vi "auton_exec.vi"(8 "test (devel auton)":bool, 9 "reinit":bool, 10 "bus_inputs":T1, 11 "bus_state":T2) -> (2 "bus_inputs out":T1, 3 "bus_state out":T2)   [LabVIEW 2013]
uses:
  structures/bus_state.ctl
  structures/bus_state_drivetrain.ctl
  structures/bus_state_collector.ctl
  collector/collector_shot_cal.ctl
  structures/bus_inputs.ctl
  auto_data.vi
  scriptlib/NAV_DRIVE_STOP.vi
  scriptlib/FIRE.vi
  scriptlib/WAIT_FOR_GUN.vi
  scriptlib/WAIT.vi
  scriptlib/NAV_DRIVE_STRAIGHT.vi
  scriptlib/CLOSE.vi
  scriptlib/WAIT_FOR_BALL.vi
  scriptlib/CAL_SET_SHOT_AUTON_1.vi
  scriptlib/SUCK.vi
  scriptlib/NOSUCK.vi
panel:
  out "autontime":u32
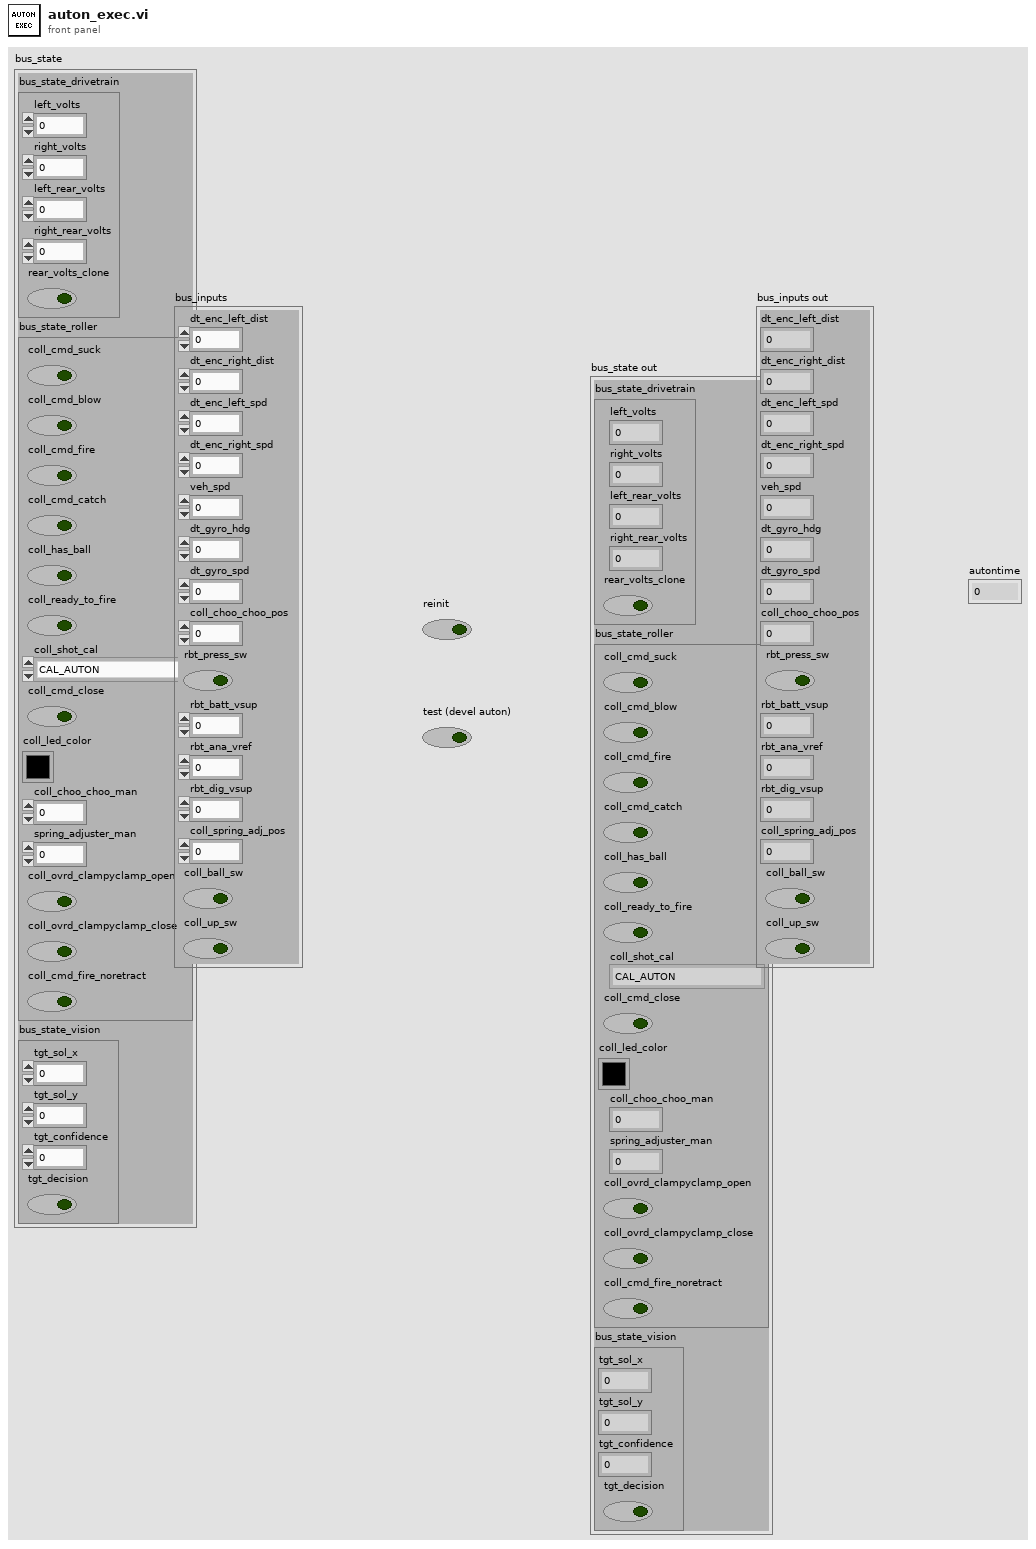
[diagram p1: front panel]
types:
  T1 = typedef "bus_inputs.ctl" = cluster{"dt_enc_left_dist":sgl, "dt_enc_right_dist":sgl, "dt_enc_left_spd":sgl, "dt_enc_right_spd":sgl, "veh_spd":sgl, "dt_gyro_hdg":sgl, "dt_gyro_spd":sgl, "coll_choo_choo_pos":sgl, "rbt_press_sw":bool, "rbt_batt_vsup":sgl, "rbt_ana_vref":dbl, "rbt_dig_vsup":dbl, "coll_spring_adj_pos":sgl, "coll_ball_sw":bool, "coll_up_sw":bool}
  T2 = typedef "bus_state.ctl" = cluster{"bus_state_drivetrain":T3, "bus_state_roller":T4, "bus_state_vision":cluster{"tgt_sol_x":dbl, "tgt_sol_y":dbl, "tgt_confidence":dbl, "tgt_decision":bool}}
  T3 = typedef "bus_state_drivetrain.ctl" = cluster{"left_volts":sgl, "right_volts":sgl, "left_rear_volts":sgl, "right_rear_volts":sgl, "rear_volts_clone":bool}
  T4 = typedef "bus_state_collector.ctl" = cluster{"coll_cmd_suck":bool, "coll_cmd_blow":bool, "coll_cmd_fire":bool, "coll_cmd_catch":bool, "coll_has_ball":bool, "coll_ready_to_fire":bool, "coll_shot_cal":T5, "coll_cmd_close":bool, "coll_led_color":u32, "coll_choo_choo_man":sgl, "spring_adjuster_man":sgl, "coll_ovrd_clampyclamp_open":bool, "coll_ovrd_clampyclamp_close":bool, "coll_cmd_fire_noretract":bool}
  T5 = typedef "collector_shot_cal.ctl" = enum16{"CAL_AUTON", "CAL_CLOSE", "CAL_MID", "CAL_FAR", "NOT_SAFE_TO_ACTUATE"}
  T6 = typedef "vi_execute.ctl" = cluster{"arguments":string[], "command":string, "refnum valid check":bool, "vi_ind":u8}
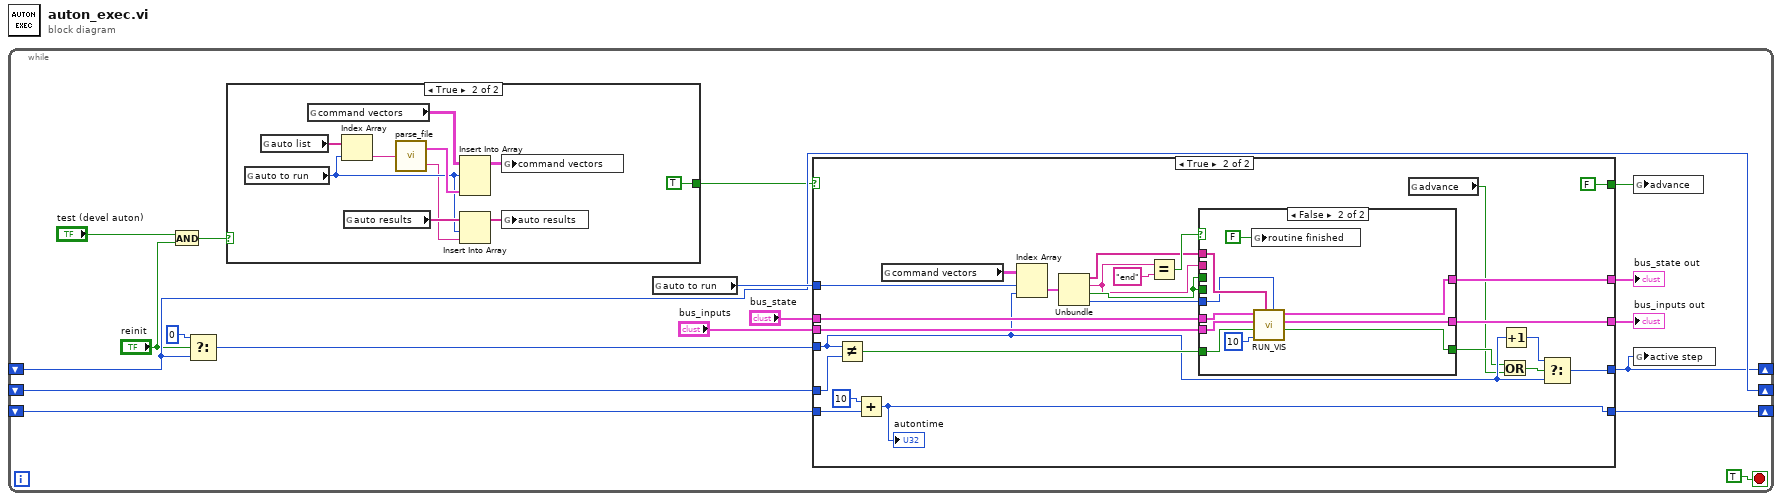
[diagram p0: block diagram]
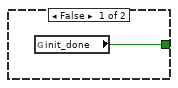
[diagram p2: hidden frame]
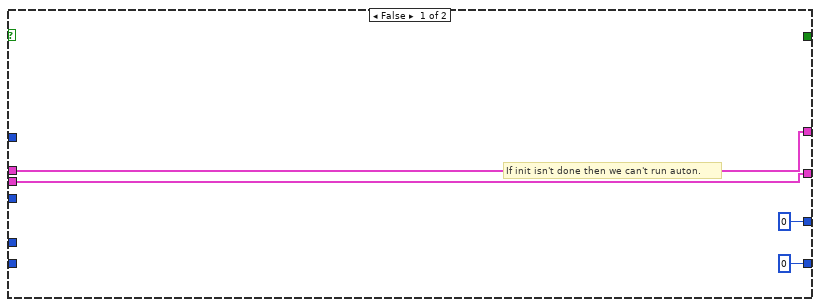
[diagram p3: hidden frame]
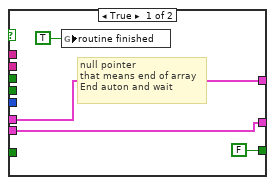
[diagram p4: hidden frame]
diagram:
  n1 = while {
    shift-right: [w2] -> _
    shift-left: _ -> [w11]
    shift-right: [w11] -> _
    shift-left: _ -> [w12]
    shift-right: [w4] -> _
    shift-left: _ -> [w5]
    stop <- TRUE stop-if-true
    n2 = And(x="test (devel auton)", y="reinit") -> (x .and. y?=w6:bool)
    n3 = Select(t=u16 0, s="reinit", f=w11) -> (s? t:f=w10:u16)
    n4 = case shown="True" w6 {
      tunnel: [w19 TRUE ("init_done")] -> w3
      frame False {
        n5 = global read "auto_data.vi" "init_done"() -> (w19:bool)
      }
      frame True {
        n6 = global read "auto_data.vi" "auto to run"() -> (w22:u8)
        n7 = global read "auto_data.vi" "auto list"() -> (w29:string[])
        n8 = global read "auto_data.vi" "command vectors"() -> (w27:T6[][])
        n9 = Index Array(array=w29, index=w22) -> (element=w28:string)
        n10 = global read "auto_data.vi" "auto results"() -> (w24:string[])
        n11 = call "parse_file.vi"("File Name With Extension"=w28) -> ("command vector"=w26:T6[], "file_status"=w21:string)
        n12 = Insert Into Array(array=w27, index (row)=w22, new element=w26) -> (w25:T6[][])  [unwired: 1 in]
        n13 = Insert Into Array(array=w24, index=w22, new element=w21) -> (w23:string[])
        n14 = global write "auto_data.vi" "command vectors"(w25) -> ()
        n15 = global write "auto_data.vi" "auto results"(w23) -> ()
      }
    }
    n16 = global read "auto_data.vi" "auto to run"() -> (w17:u8)
    n17 = case shown="True" w3 {
      tunnel: w17 -> [_ w43]
      tunnel: w10 -> [_ w42]
      tunnel: "bus_state" -> [w33 w54]
      tunnel: [w33 w56] -> w15
      tunnel: [w32 w55] -> w14
      tunnel: "bus_inputs" -> [w32 w53]
      tunnel: [u16 0 w50] -> w2
      tunnel: w12 -> [_ w52]
      tunnel: w5 -> [_ w48]
      tunnel: [u32 0 w47] -> w4
      tunnel: [_ FALSE] -> w1
      frame False {
        # "If init isn't done then we can't run auton."
      }
      frame True {
        n18 = Not Equal?(x=w42, y=w52) -> (x != y?=w51:bool)
        n19 = Add(x=u32 10, y=w48) -> (x+y=w47:u32)
        "autontime" <- w47
        n20 = global read "auto_data.vi" "command vectors"() -> (w58:T6[][])
        n21 = Index Array(array=w58, index (row)=w43, index (col)=w42) -> (element=w57:T6)
        n22 = Unbundle(w57) -> ("arguments"=w44:string[], "command"=w35:string, "refnum valid check"=w37:bool, "vi_ind"=w36:u8)
        n23 = Equal?(x=w35, y="end") -> (x = y?=w45:bool)
        n24 = case shown="False" w45 {
          tunnel: w44 -> [_ w70]
          tunnel: w35 -> [_ _]
          tunnel: [w62 w66] -> w56
          tunnel: [w60 w65] -> w55
          tunnel: w54 -> [w62 w71]
          tunnel: w53 -> [w60 w67]
          tunnel: w51 -> [_ w68]
          tunnel: [FALSE ("Done") w64] -> w40
          tunnel: w37 -> [_ _]
          tunnel: w37 -> [_ _]
          tunnel: w36 -> [_ w63]
          frame True {
            # "null pointer\nthat means end of array\nEnd auton and wait"
            n25 = global write "auto_data.vi" "routine finished"(TRUE ("routine finished")) -> ()
          }
          frame False {
            n26 = global write "auto_data.vi" "routine finished"(FALSE ("routine finished")) -> ()
            n27 = call "RUN_VIS.vi"("index"=w63, "arguments"=w70, "dt"=10, "Reinit"=w68, "bus_inputs"=w67, "bus_state"=w71) -> ("Done"=w64:bool, "bus_inputs out"=w65:T1, "bus_state out"=w66:T2)  [unwired: 3 in]
          }
        }
        n28 = global read "auto_data.vi" "advance"() -> (w38:bool)
        n29 = Or(x=w40, y=w38) -> (x .or. y?=w39:bool)
        n30 = Increment(x=w42) -> (x+1=w49:u16)
        n31 = Select(t=w49, s=w39, f=w42) -> (s? t:f=w50:u16)
      }
    }
    "bus_state out" <- w15
    "bus_inputs out" <- w14
    n32 = global write "auto_data.vi" "advance"(w1) -> ()
    n33 = global write "auto_data.vi" "active step"(w2) -> ()
  }
